vi "FTW-Router-Destroy.vi"(0 "FTW Router":refnum<class "FTW-Router.lvclass">, 11 "error in":errorcluster) -> (15 "error out":errorcluster)   [LabVIEW 2013, in "FTW-Router.lvclass"]
uses:
  FTW-Router.lvclass
  FTW-Router.lvclass/FTW-Router.ctl
  socket/FTW-Socket.lvclass
panel:
  # "Inputs"
  # "Outputs"
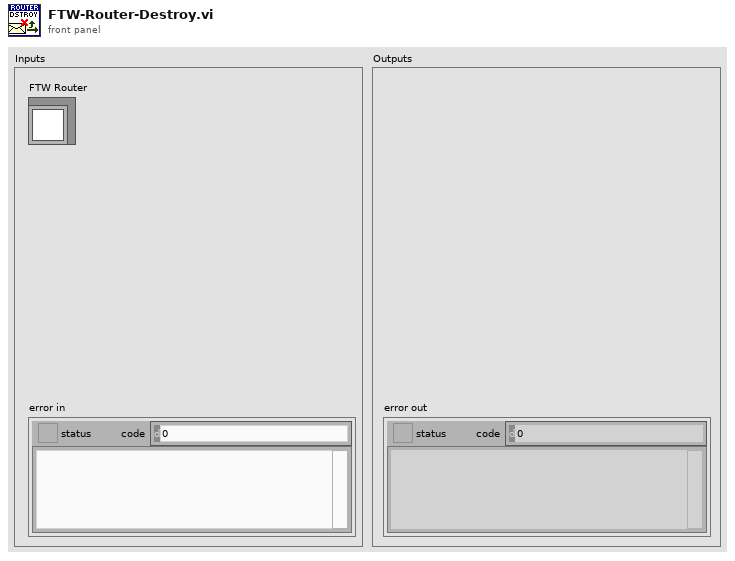
[diagram p1: front panel]
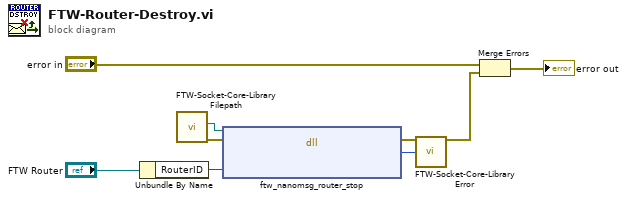
[diagram p0: block diagram]
diagram:
  n1 = Unbundle By Name("FTW Router") -> ("RouterID"=w1:i64)
  n2 = call "FTW-Socket-Core-LibraryFilepath.vi"() -> ("error out"=w2:errorcluster, "Library Filepath"=w5:path)  [unwired: 9 in, 1 out]
  n3 = dll-call lib="C:/Users/Jack/repo/ftw-master/Actor/src/Endpoint/Core/FTWLib-nanomsg32.dll" fn="ftw_nanomsg_router_stop"(path in=w5, error in=w2, "RouterID"=w1) -> (error out=w4:errorcluster, "Return Value"=w3:i64)  [unwired: 2 in, 1 out]
  n4 = call "FTW-Socket-Core-LibraryError.vi"("error in"=w4, "Return Value"=w3) -> ("error out"=w8:errorcluster)  [unwired: 13 in]
  n5 = Merge Errors("error in", w8) -> (→"error out":errorcluster)
